vi "Auto Match.vi"() -> ()   [LabVIEW 2014]
panel:
  out "# of Iterations":i32
  out "Current Number":dbl
  in  "Number to Match":dbl=50.0 min=0.0 max=1000.0 step=1.0 format="%#.0f"
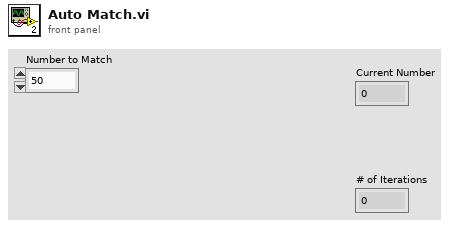
[diagram p1: front panel]
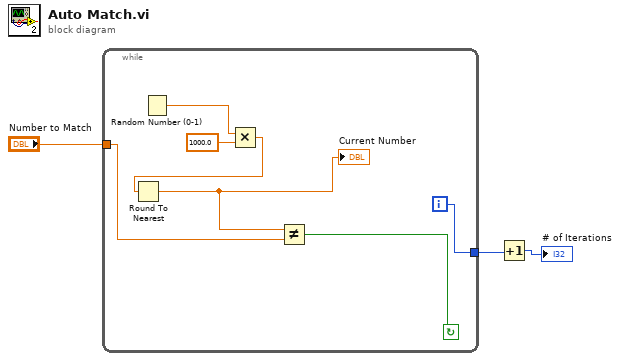
[diagram p0: block diagram]
diagram:
  n1 = while {
    tunnel: "Number to Match" -> [w6]
    tunnel: [w4] -> w2
    i -> [w4]
    stop <- w5 continue-if-true
    n2 = Random Number (0-1)() -> (number: 0 to 1=w10:dbl)
    n3 = Multiply(x=w10, y=1000.0) -> (x*y=w8:dbl)
    n4 = Round To Nearest(number=w8) -> (nearest integer value=w7:dbl)
    "Current Number" <- w7
    n5 = Not Equal?(x=w7, y=w6) -> (x != y?=w5:bool)
  }
  n6 = Increment(x=w2) -> (x+1=→"# of Iterations":i32)
